vi "sub_Force_Sensor_data.vi"(7 "cmd":enum16{"write", "read"}(ring), 11 "Force Sensor data":T1) -> (3 "Force Sensor data out":T1)   [LabVIEW 2016]
uses:
  ctl/force_sensor_data.ctl
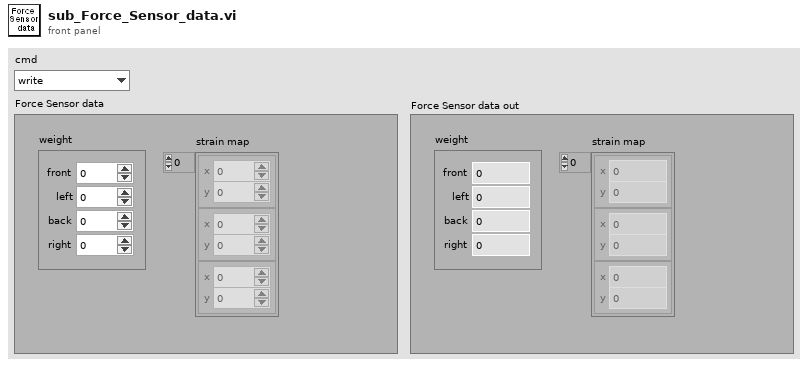
[diagram p1: front panel]
types:
  T1 = typedef "force_sensor_data.ctl" = cluster{"weight":cluster{"front":dbl, "left":dbl, "back":dbl, "right":dbl}, "strain map":cluster{"x":dbl, "y":dbl}[]}
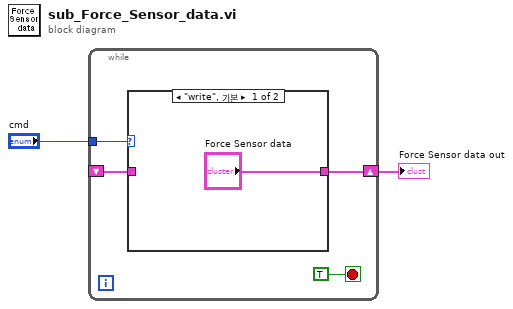
[diagram p0: block diagram]
diagram:
  n1 = while {
    shift-right: [w4] -> w1
    shift-left: _ -> [w3]
    tunnel: "cmd" -> [w5]
    stop <- TRUE stop-if-true
    n2 = case shown="\"write\", 기본" w5 {
      tunnel: ["Force Sensor data" w8] -> w4
      tunnel: w3 -> [_ w8]
      frame "write", Default {
      }
      frame "read" {
      }
    }
  }
  "Force Sensor data out" <- w1
